vi "IO test.vi"() -> ()   [LabVIEW 2015]
panel:
  out "input":dynamicdata(graph)
  in  "stop":bool
  in  "amplitude":dbl
  out "output":dynamicdata(graph)
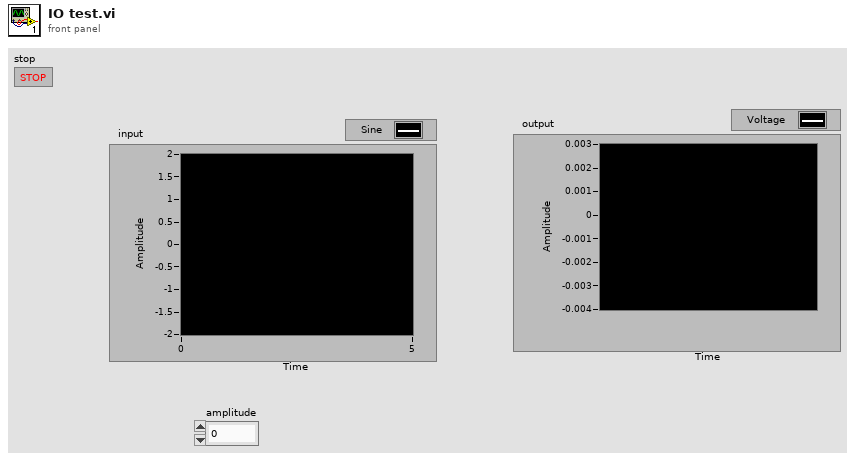
[diagram p1: front panel]
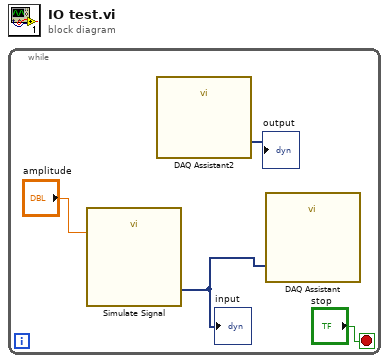
[diagram p0: block diagram]
diagram:
  n1 = while {
    stop <- "stop" stop-if-true
    n2 = call "Simulate Signal"("Amplitude"="amplitude") -> ("Sine"=w1:dynamicdata)  [unwired: 13 in, 1 out]
    "input" <- w1
    n3 = call "DAQ Assistant2"() -> ("data"=→"output":dynamicdata)  [unwired: 17 in, 2 out]
    n4 = call "DAQ Assistant"("data"=w1) -> ()  [unwired: 17 in, 2 out]
  }
